vi "Does It Fit.vi"(9 "Inner Rect":T1, 10 "Outer Rect":T1) -> (2 "Fit?":bool)   [LabVIEW 2012, in "String XControl.xctl"]
uses:
  String XControl.xctl
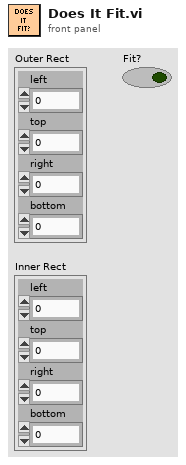
[diagram p1: front panel]
types:
  T1 = cluster{"left":i16, "top":i16, "right":i16, "bottom":i16}
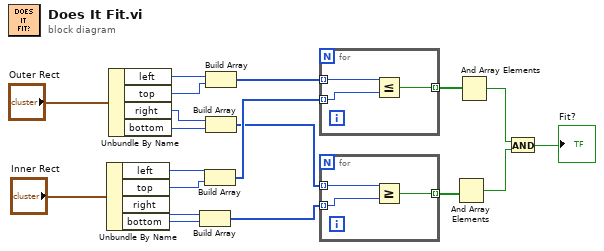
[diagram p0: block diagram]
diagram:
  n1 = Unbundle By Name("Inner Rect") -> ("left"=w13:i16, "top"=w12:i16, "right"=w11:i16, "bottom"=w10:i16)
  n2 = Unbundle By Name("Outer Rect") -> ("left"=w17:i16, "top"=w16:i16, "right"=w15:i16, "bottom"=w14:i16)
  n3 = Build Array(w11, w10) -> (w6:i16[])
  n4 = Build Array(w13, w12) -> (w8:i16[])
  n5 = Build Array(w17, w16) -> (w9:i16[])
  n6 = Build Array(w15, w14) -> (w7:i16[])
  n7 = for {
    tunnel: w9 -> [w22] mode=indexing
    tunnel: w8 -> [w21] mode=indexing
    tunnel: [w20] -> w5 mode=indexing
    n8 = Less Or Equal?(x=w22, y=w21) -> (x <= y?=w20:bool)
  }
  n9 = for {
    tunnel: w7 -> [w25] mode=indexing
    tunnel: w6 -> [w24] mode=indexing
    tunnel: [w23] -> w4 mode=indexing
    n10 = Greater Or Equal?(x=w25, y=w24) -> (x >= y?=w23:bool)
  }
  n11 = And Array Elements(Boolean array=w4) -> (logical AND=w2:bool)
  n12 = And Array Elements(Boolean array=w5) -> (logical AND=w3:bool)
  n13 = And(x=w3, y=w2) -> (x .and. y?=→"Fit?":bool)
